vi "VISA Close.vi"(8 "error in (no error)":errorcluster, 11 "VISA In":refnum<visa-resource-name>) -> (0 "error out":errorcluster)   [LabVIEW 2014, in "VISA.lvlib"]
uses:
  VISA.lvlib
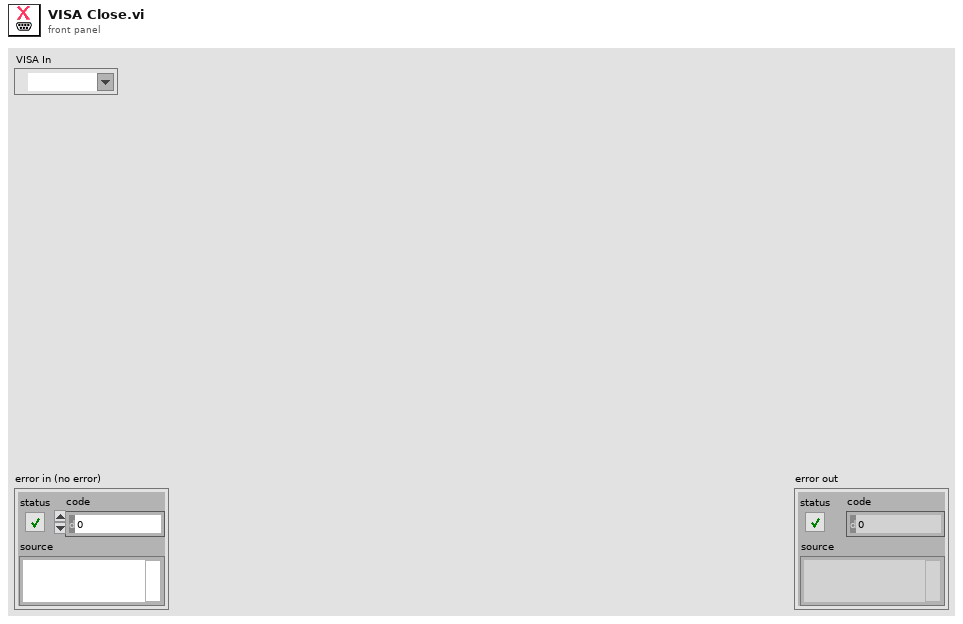
[diagram p1: front panel]
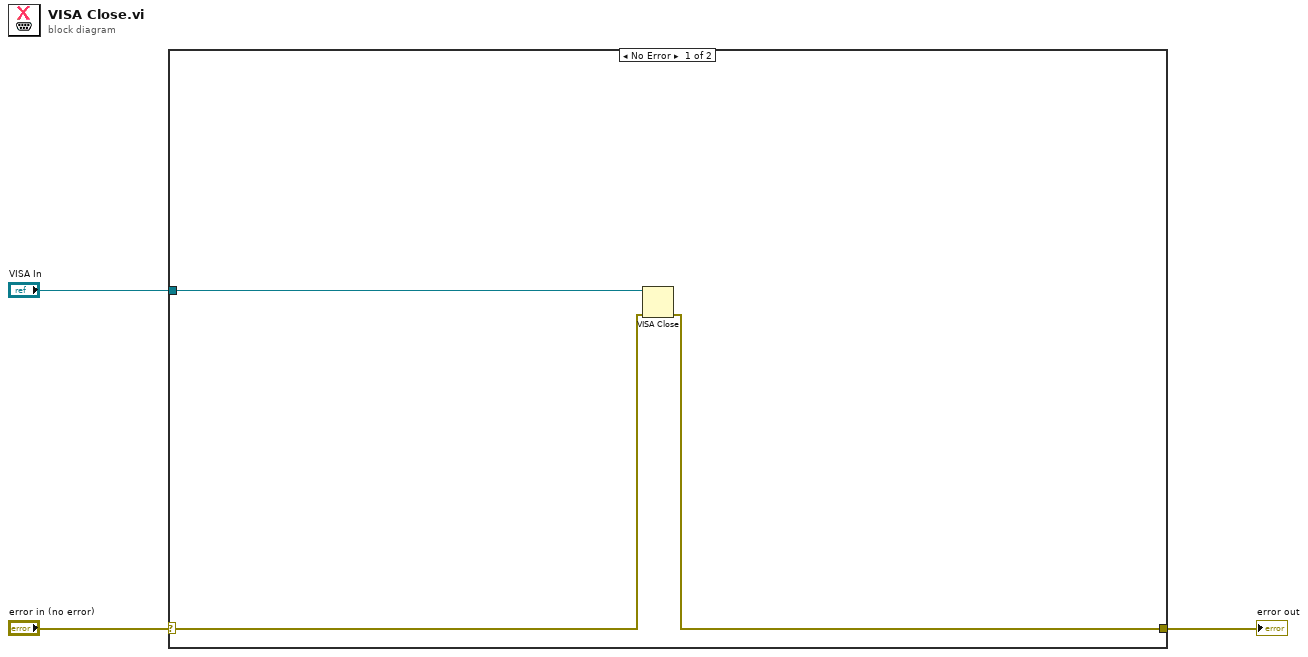
[diagram p0: block diagram]
diagram:
  n1 = case shown="No Error" "error in (no error)" {
    selector: "error in (no error)" -> [w6 w7]
    tunnel: [w5 w7] -> w2
    tunnel: "VISA In" -> [w4 _]
    frame No Error {
      n2 = VISA Close(VISA resource name=w4, error in (no error)=w6) -> (error out=w5:errorcluster)
    }
    frame Error {
    }
  }
  "error out" <- w2
